vi "Configure Event Log.vi"(5 "Log Number (1: No 1)":i32(ring)=1 items=["No 1"=1, "No 2"=2, "No 3"=3, "No 4"=4], 6 "Log Message (\"\")":string, 7 "Log Level (0: Info)":i32(ring) items=["Info", "Warning", "Error"], 8 "error in (no error)":errorcluster, 10 "Block Number (1)":u32=1, 11 "VISA resource name":refnum<visa-resource-name>) -> (0 "error out":errorcluster, 3 "VISA resource name out":refnum<visa-resource-name>)   [LabVIEW 2015, in "Keithley DMM6500 DAQ6500 Series.lvlib"]
doc: "Allows you to log an event in the event log when the trigger model is running."
uses:
  <instrlib>/Keithley DMM6500 DAQ6500 Series/Keithley DMM6500 DAQ6500 Series.lvlib
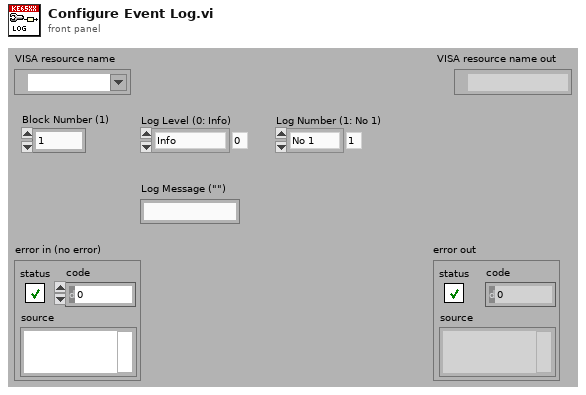
[diagram p1: front panel]
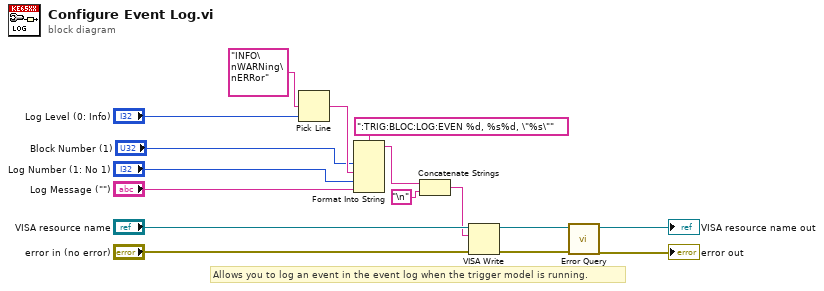
[diagram p0: block diagram]
diagram:
  # "Allows you to log an event in the event log when the trigger model is running."
  n1 = Pick Line(multi-line string="INFO\nWARNing\nERRor", line index="Log Level (0: Info)") -> (output string=w8:string)  [unwired: 1 in]
  n2 = Format Into String(format string=":TRIG:BLOC:LOG:EVEN %d, %s%d, \"%s\"", "Block Number (1)", w8, "Log Number (1: No 1)", "Log Message (\"\")") -> (resulting string=w4:string)  [unwired: 2 in, 1 out]
  n3 = Concatenate Strings(w4, "\n") -> (w5:string)
  n4 = VISA Write(VISA resource name="VISA resource name", write buffer=w5, error in (no error)="error in (no error)") -> (VISA resource name out=w12:refnum<visa-resource-name>, error out=w11:errorcluster)  [unwired: 1 out]
  n5 = call <instrlib>:"Error Query.vi"("error in (no error)"=w11, "VISA resource name"=w12) -> ("error out"=→"error out":errorcluster, "VISA resource name out"=→"VISA resource name out":refnum<visa-resource-name>)  [unwired: 6 in, 2 out]
